vi "level mansurment.vi"() -> ()   [LabVIEW 2015]
panel:
  in  "stop":bool
  out "Meter":dbl(knob) scale=0.0..20.0
  out "Tank":dbl(slide) scale=300.0..500.0
  in  "Numeric 3":dbl
  in  "Numeric 2":dbl
  in  "Slide":dbl(slide) scale=0.0..10.0
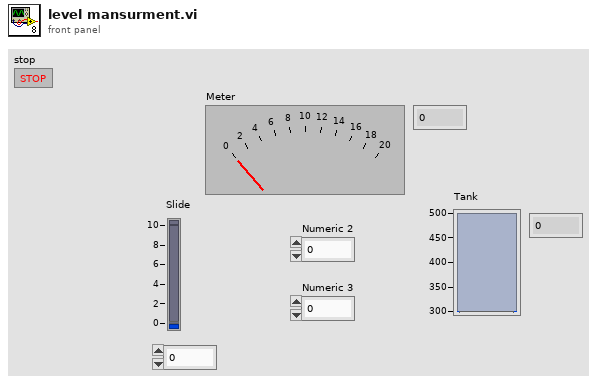
[diagram p1: front panel]
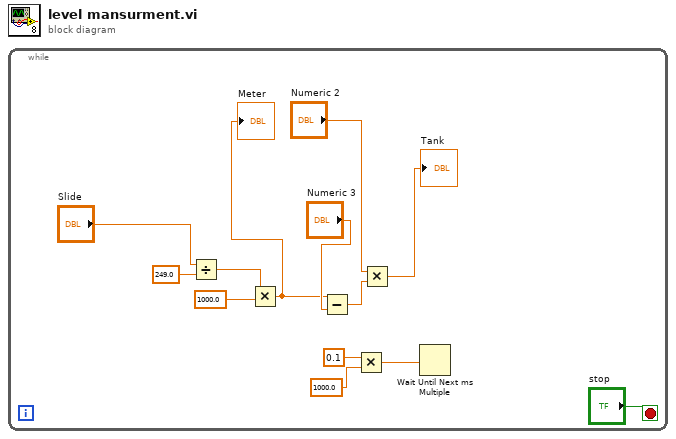
[diagram p0: block diagram]
diagram:
  n1 = while {
    stop <- "stop" stop-if-true
    n2 = Divide(x="Slide", y=249.0) -> (x/y=w11:dbl)
    n3 = Multiply(x=w11, y=1000.0) -> (x*y=w1:dbl)
    "Meter" <- w1
    n4 = Subtract(x=w1, y="Numeric 3") -> (x-y=w8:dbl)
    n5 = Multiply(x=0.1, y=1000.0) -> (x*y=w2:dbl)
    n6 = Multiply(x="Numeric 2", y=w8) -> (x*y=→"Tank":dbl)
    n7 = Wait Until Next ms Multiple(millisecond multiple=w2) -> ()  [unwired: 1 out]
  }
